vi "create imaq images.vi"(8 "error in (no error)":errorcluster, 11 "Thorcam in":refnum<class "Thorcam.lvclass">) -> (0 "error out":errorcluster, 3 "Thorcam out":refnum<class "Thorcam.lvclass">)   [LabVIEW 2012, in "Thorcam.lvclass"]
uses:
  Thorcam.lvclass
  Thorcam.lvclass/Thorcam.ctl
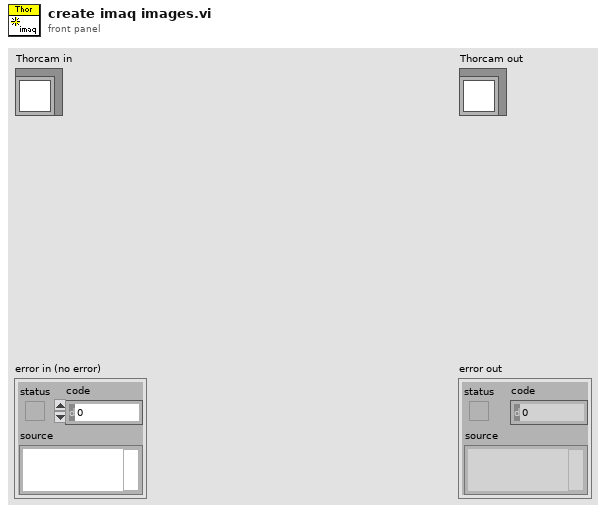
[diagram p1: front panel]
types:
  T1 = typedef "Image Type" = u32
  T2 = typedef "IMAQ Image.ctl" = refnum<image>
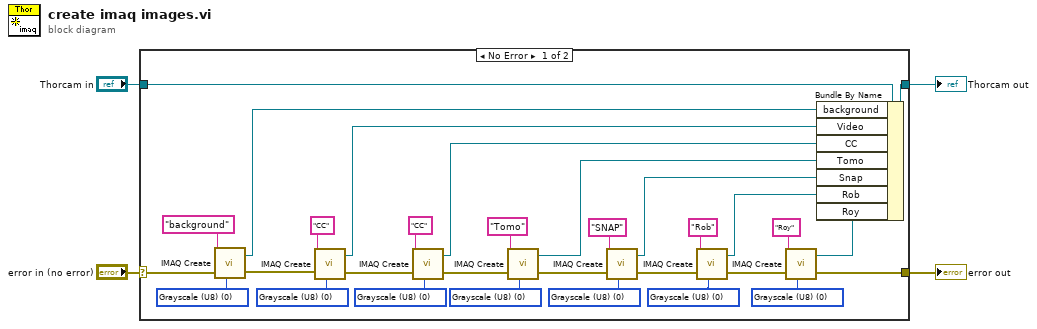
[diagram p0: block diagram]
diagram:
  n1 = case shown="No Error" "error in (no error)" {
    selector: "error in (no error)" -> [w7 w37]
    tunnel: [w33 w37] -> w3
    tunnel: [w28 w36] -> w1
    tunnel: "Thorcam in" -> [w29 w36]
    frame No Error {
      w8 = T1 0 items=["Grayscale (U8)", "Grayscale (I16)", "Grayscale (SGL)", "Complex (CSG)", "RGB (U32)", "HSL (U32)", "RGB (U64)", "Grayscale (U16)"] ("Image Type")
      w13 = T1 0 items=["Grayscale (U8)", "Grayscale (I16)", "Grayscale (SGL)", "Complex (CSG)", "RGB (U32)", "HSL (U32)", "RGB (U64)", "Grayscale (U16)"] ("Image Type")
      w17 = T1 0 items=["Grayscale (U8)", "Grayscale (I16)", "Grayscale (SGL)", "Complex (CSG)", "RGB (U32)", "HSL (U32)", "RGB (U64)", "Grayscale (U16)"] ("Image Type")
      w16 = T1 0 items=["Grayscale (U8)", "Grayscale (I16)", "Grayscale (SGL)", "Complex (CSG)", "RGB (U32)", "HSL (U32)", "RGB (U64)", "Grayscale (U16)"] ("Image Type")
      w25 = T1 0 items=["Grayscale (U8)", "Grayscale (I16)", "Grayscale (SGL)", "Complex (CSG)", "RGB (U32)", "HSL (U32)", "RGB (U64)", "Grayscale (U16)"] ("Image Type")
      w26 = T1 0 items=["Grayscale (U8)", "Grayscale (I16)", "Grayscale (SGL)", "Complex (CSG)", "RGB (U32)", "HSL (U32)", "RGB (U64)", "Grayscale (U16)"] ("Image Type")
      w27 = T1 0 items=["Grayscale (U8)", "Grayscale (I16)", "Grayscale (SGL)", "Complex (CSG)", "RGB (U32)", "HSL (U32)", "RGB (U64)", "Grayscale (U16)"] ("Image Type")
      n2 = call "IMAQ Create"("Image Name"="background", "Image Type"=w8, "error in (no error)"=w7) -> ("New Image"=w5:T2, "error out"=w6:errorcluster)  [unwired: 2 in]
      n3 = call "IMAQ Create"("Image Name"="CC", "Image Type"=w13, "error in (no error)"=w6) -> ("New Image"=w10:T2, "error out"=w11:errorcluster)  [unwired: 2 in]
      n4 = call "IMAQ Create"("Image Name"="CC", "Image Type"=w17, "error in (no error)"=w11) -> ("New Image"=w14:T2, "error out"=w19:errorcluster)  [unwired: 2 in]
      n5 = call "IMAQ Create"("Image Name"="Tomo", "Image Type"=w16, "error in (no error)"=w19) -> ("New Image"=w15:T2, "error out"=w18:errorcluster)  [unwired: 2 in]
      n6 = call "IMAQ Create"("Image Name"="SNAP", "Image Type"=w27, "error in (no error)"=w18) -> ("New Image"=w24:T2, "error out"=w35:errorcluster)  [unwired: 2 in]
      n7 = call "IMAQ Create"("Image Name"="Rob", "Image Type"=w26, "error in (no error)"=w35) -> ("New Image"=w23:T2, "error out"=w34:errorcluster)  [unwired: 2 in]
      n8 = call "IMAQ Create"("Image Name"="Roy", "Image Type"=w25, "error in (no error)"=w34) -> ("New Image"=w22:T2, "error out"=w33:errorcluster)  [unwired: 2 in]
      n9 = Bundle By Name(cluster=w29, "background"=w5, "Video"=w10, "CC"=w14, "Tomo"=w15, "Snap"=w24, "Rob"=w23, "Roy"=w22) -> (w28:refnum<class "Thorcam.lvclass">)
    }
    frame Error {
    }
  }
  "error out" <- w3
  "Thorcam out" <- w1
